vi "Create.vi"(8 "Error In":errorcluster, 11 "Reader":refnum<class "Reader.lvclass">) -> (0 "Error Out":errorcluster, 3 "Parser":refnum<class "Parser.lvclass">)   [LabVIEW 2017, in "Mustache.lvlib" / "Parser.lvclass"]
uses:
  Parser.lvclass
  Reader/Reader.lvclass
  Controls/States.ctl
  Parser.lvclass/Parser.ctl
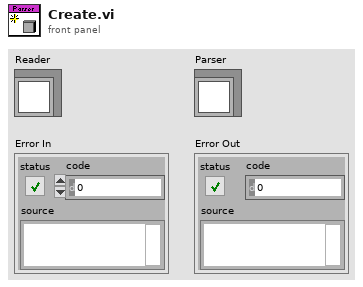
[diagram p1: front panel]
types:
  T1 = typedef "Mustache.lvlib/Parser.lvclass/States.ctl" = enum16{"Text", "Opening Tag", "Tag", "Closing Tag"}
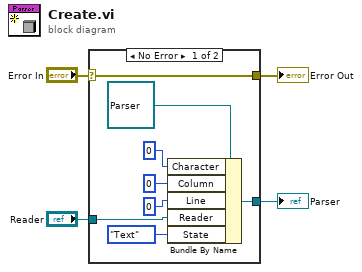
[diagram p0: block diagram]
diagram:
  n1 = case shown="No Error" "Error In" {
    selector: "Error In" -> [w11 w13]
    tunnel: [w11 w13] -> w3
    tunnel: [w5 _] -> w2
    tunnel: "Reader" -> [w10 _]
    frame No Error {
      n2 = Bundle By Name(cluster=refnum<class "Parser.lvclass"> refnum ("Mustache.lvlib:Parser.lvclass"), "Character"=u8 0, "Column"=u64 0, "Line"=u64 0, "Reader"=w10, "State"=States."Text") -> (w5:refnum<class "Parser.lvclass">)
    }
    frame Error {
    }
  }
  "Error Out" <- w3
  "Parser" <- w2
